vi "Pure Function.vi"(10 "Offset":i32, 11 "Iterations":i32) -> (3 "Output Array":i32[](array[numeric]))   [LabVIEW 2019]
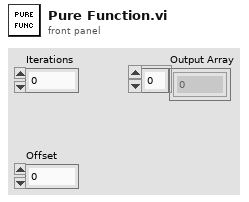
[diagram p1: front panel]
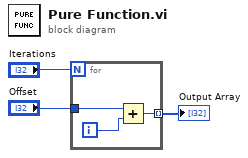
[diagram p0: block diagram]
diagram:
  n1 = for {
    N: "Iterations" -> [_]
    tunnel: "Offset" -> [w6]
    tunnel: [w4] -> w1 mode=indexing
    i -> [w5]
    n2 = Add(x=w6, y=w5) -> (x+y=w4:i32)
  }
  "Output Array" <- w1
